vi "snmpset_int.vi"(7 "value":i32, 8 "error in (no error)":errorcluster, 9 "OID":string=".1.3.6.1.4.1.3808.1.1.3.3.3.1.1.4.1 ", 10 "community":string="private", 11 "IP / Hostname":string="172.20.125.112") -> (0 "error out":errorcluster, 3 "return":string="1\r\n")   [LabVIEW 2021]
panel:
  out "snmpset arguments":string="-r:172.20.125.112 -c:private -o:.1.3.6.1.4.1.3808.1.1.3.3.3.1.1.4.1  -q"
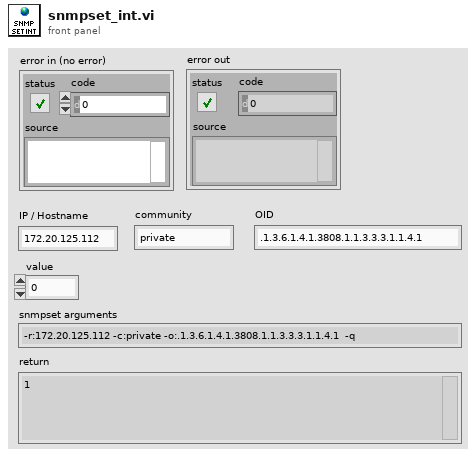
[diagram p1: front panel]
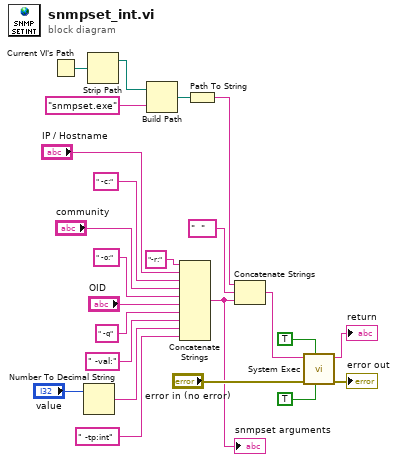
[diagram p0: block diagram]
diagram:
  n1 = Current VI's Path() -> (path=w1:path)
  n2 = Number To Decimal String(number="value") -> (decimal integer string=w4:string)  [unwired: 1 in]
  n3 = Strip Path(path=w1) -> (stripped path=w2:path)  [unwired: 1 out]
  n4 = Build Path(base path=w2, name or relative path="snmpset.exe") -> (appended path=w21:path)
  n5 = Concatenate Strings("-r:" ("string"), "IP / Hostname", " -c:" ("string"), "community", " -o:" ("string"), "OID", " -q" ("string"), " -val:" ("string"), w4, " -tp:int" ("string")) -> (w9:string)
  "snmpset arguments" <- w9
  n6 = Path To String(path=w21) -> (string=w23:string)
  n7 = Concatenate Strings(w23, "  " ("standard input"), w9) -> (w18:string)
  n8 = call <vilib>:"System Exec.vi"("run minimized? (F)"=TRUE, "wait until completion? (T)"=TRUE, "error in (no error)"="error in (no error)", "command line"=w18) -> ("error out"=→"error out":errorcluster, "standard output"=→"return":string)  [unwired: 2 in, 4 out]
